vi "UI.vi"(0 "reference in":refnum<class "GUI Setting.lvclass">, 5 "error in (no error)":errorcluster) -> (14 "reference out":refnum<class "GUI Setting.lvclass">, 19 "error out":errorcluster)   [LabVIEW 2019, in "GUI Setting.lvclass"]
uses:
  GUI Setting.lvclass
  D:/GIT H4000/H4000/src/GUI_class/GUI.lvclass
  GUI Settings Indicator.ctl
  GUI_class/GUI.lvclass/GUI.ctl
  d678bd6a-011c-496f-8712-f7d087665a22.vi
  GUI_class/Set Win State.vi
  GUI_class/protected/GetSheredData.vi
  <vilib>/Utility/error.llb/Clear Errors.vi
  ConfigInterface_class/ConfigInterface.lvclass
  GUI_class/GUI.lvclass
  SV_Wrap/SharedVariableWrapper.lvclass
panel:
  in  "GUI Settings Indicator":T1
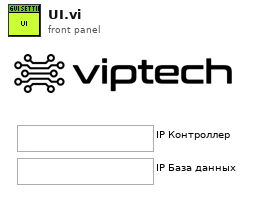
[diagram p1: front panel]
types:
  T1 = typedef "GUI Setting.lvclass/GUI Settings Indicator.ctl" = cluster{"ip_controller":string, "ip_db":string}
  T2 = enum32{"Invalid", "Standard", "Closed", "Hidden", "Minimized", "Maximized"}
  T3 = enum32{"invalid app kind", "Development System", "Run Time System", "Student Edition", "Embedded LabVIEW", "Evaluation", "Custom"}
  T4 = cluster{"Core":cluster{"Current VI Reference":refnum<vi>, "Close Panel on Exit?":bool}, "file settings":string, "GUI Settings Indicator":T1}
  T5 = cluster{"Current VI Reference":refnum<vi>, "Close Panel on Exit?":bool}
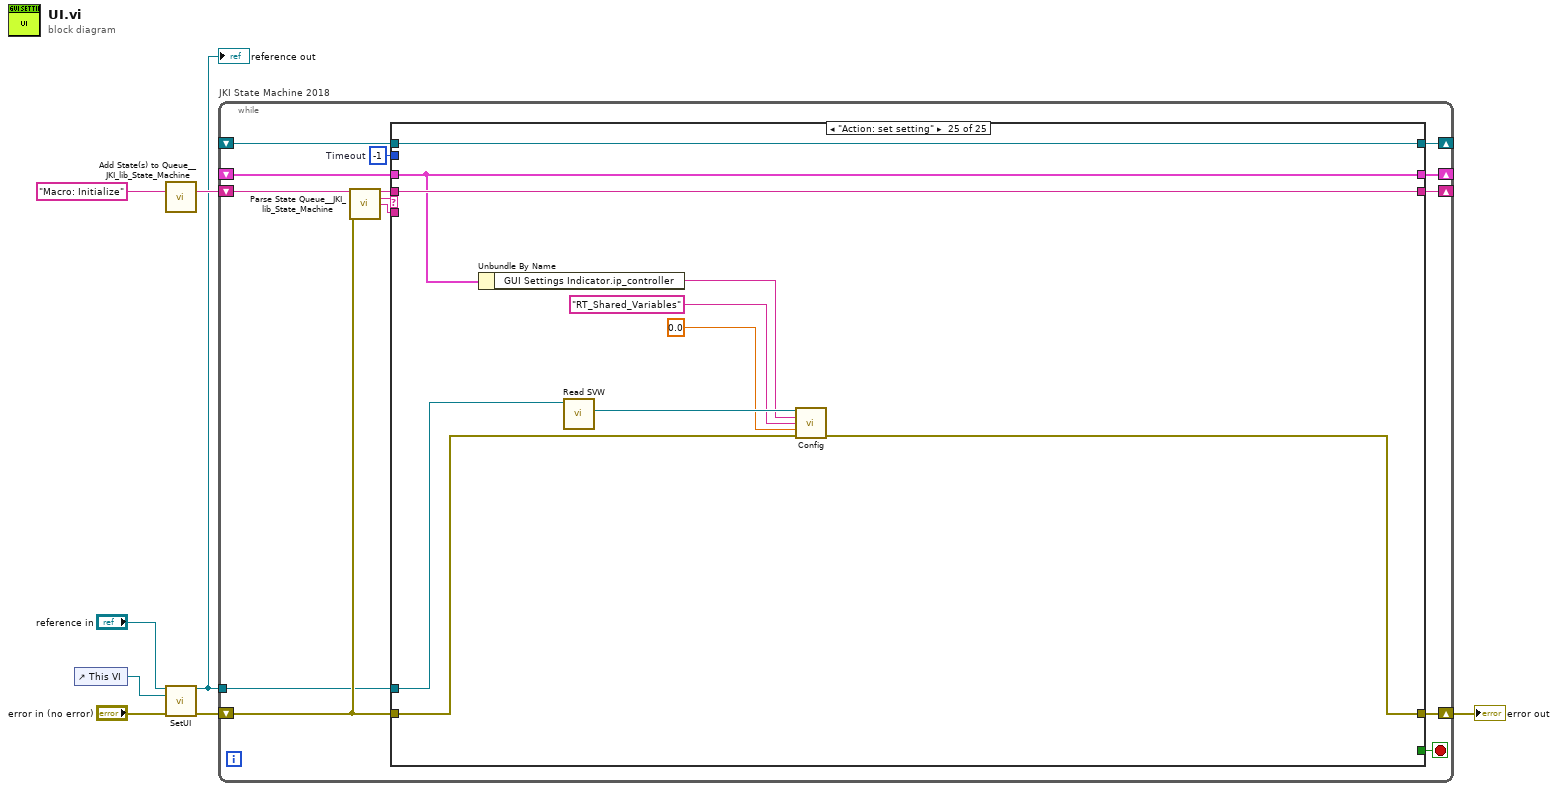
[diagram p0: block diagram]
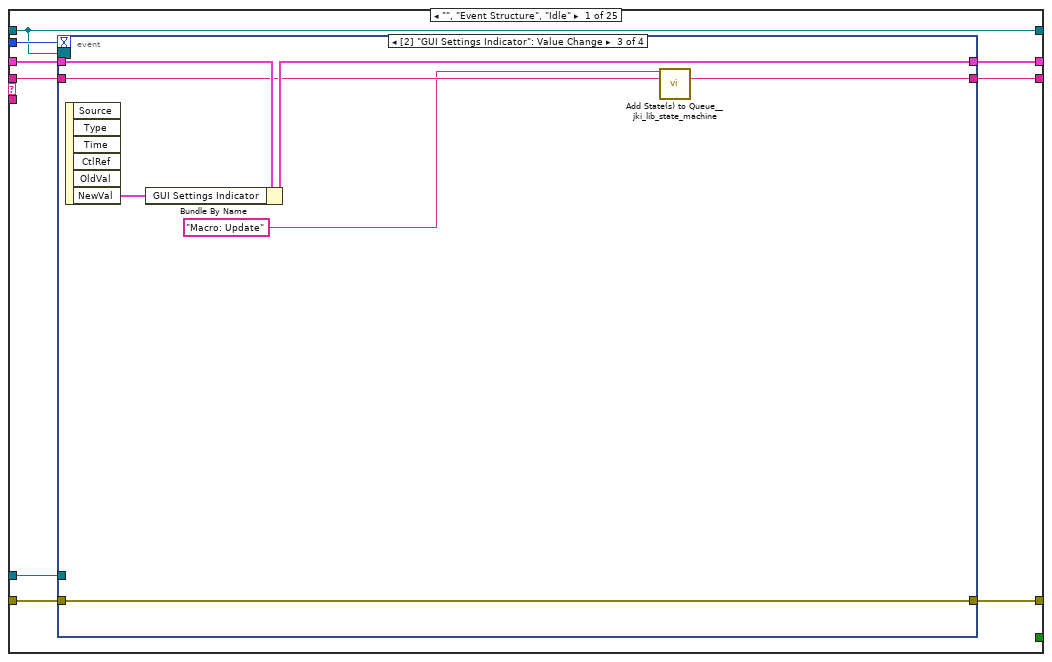
[diagram p2: hidden frame]
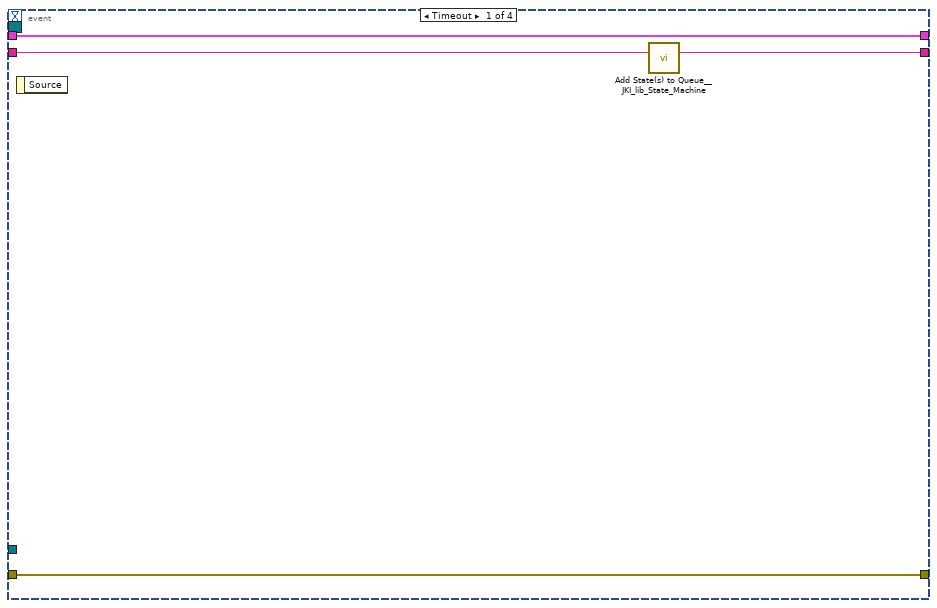
[diagram p3: hidden frame]
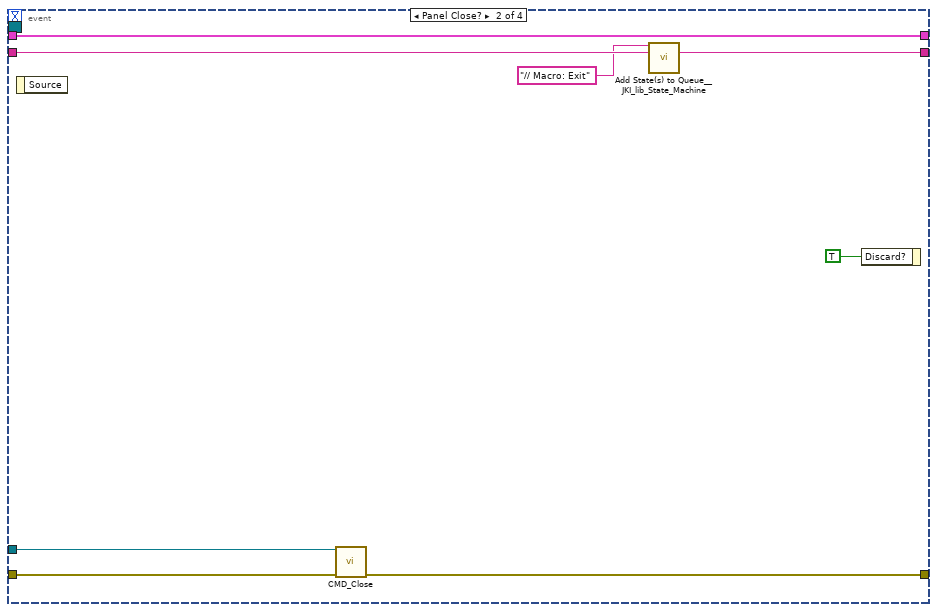
[diagram p4: hidden frame]
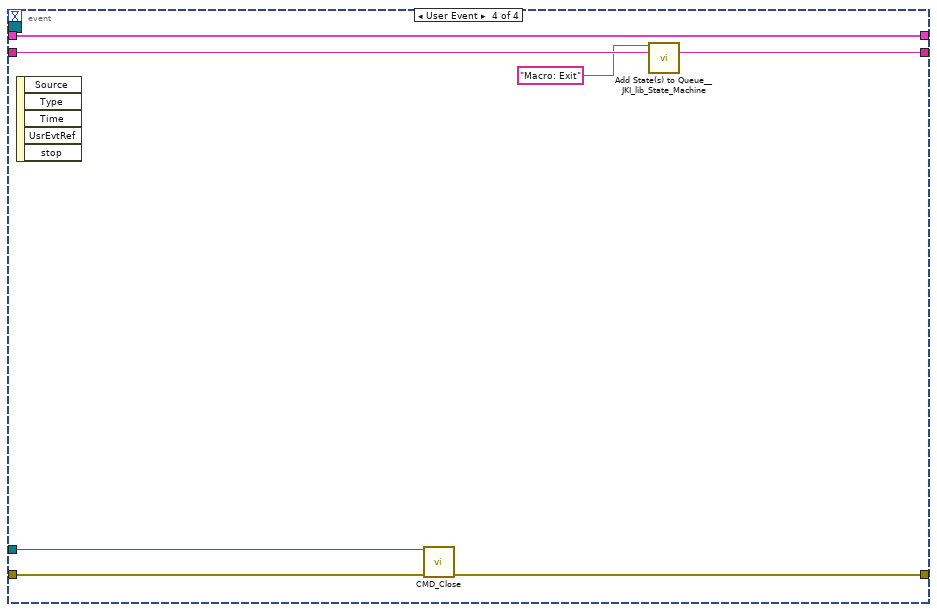
[diagram p5: hidden frame]
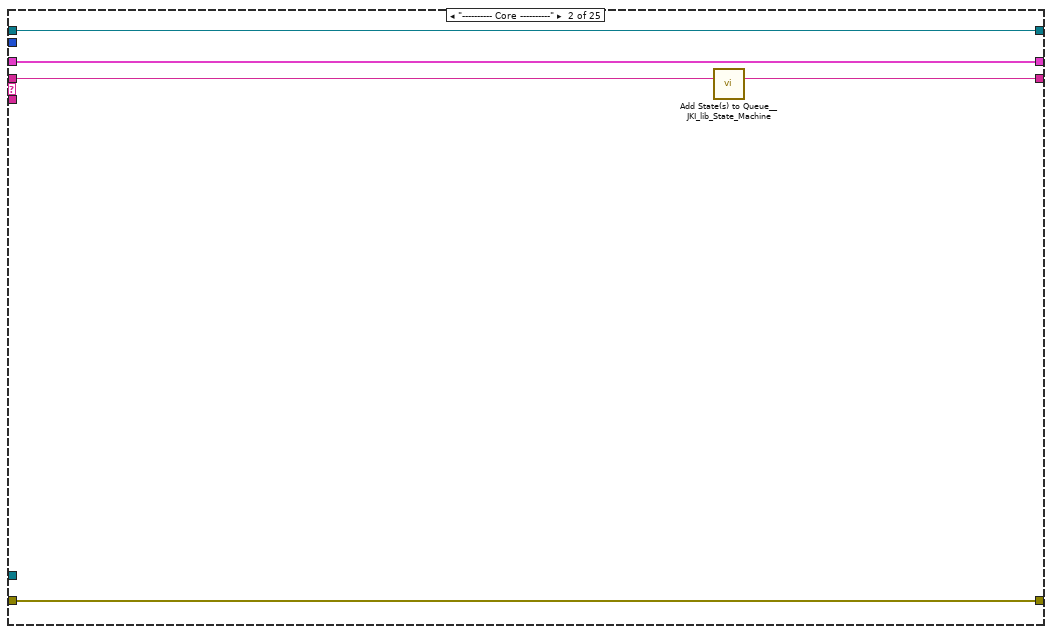
[diagram p6: hidden frame]
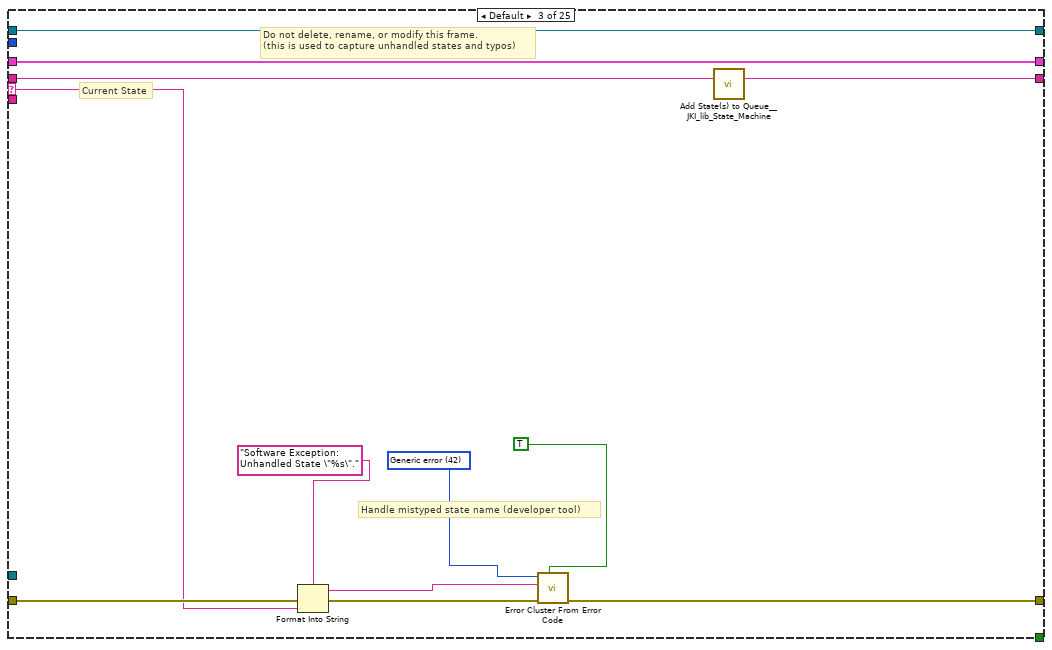
[diagram p7: hidden frame]
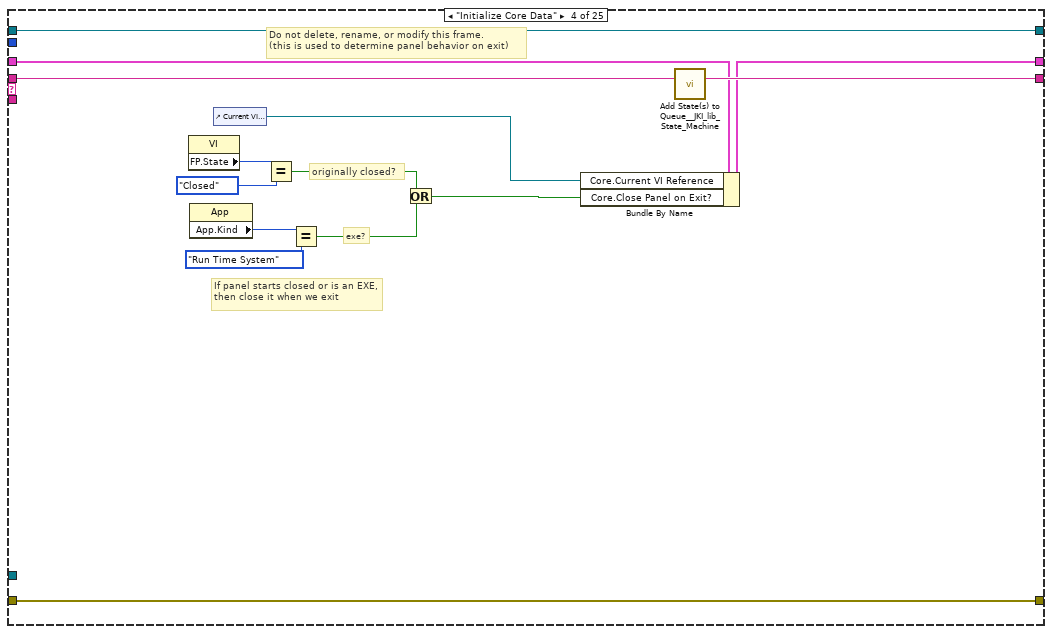
[diagram p8: hidden frame]
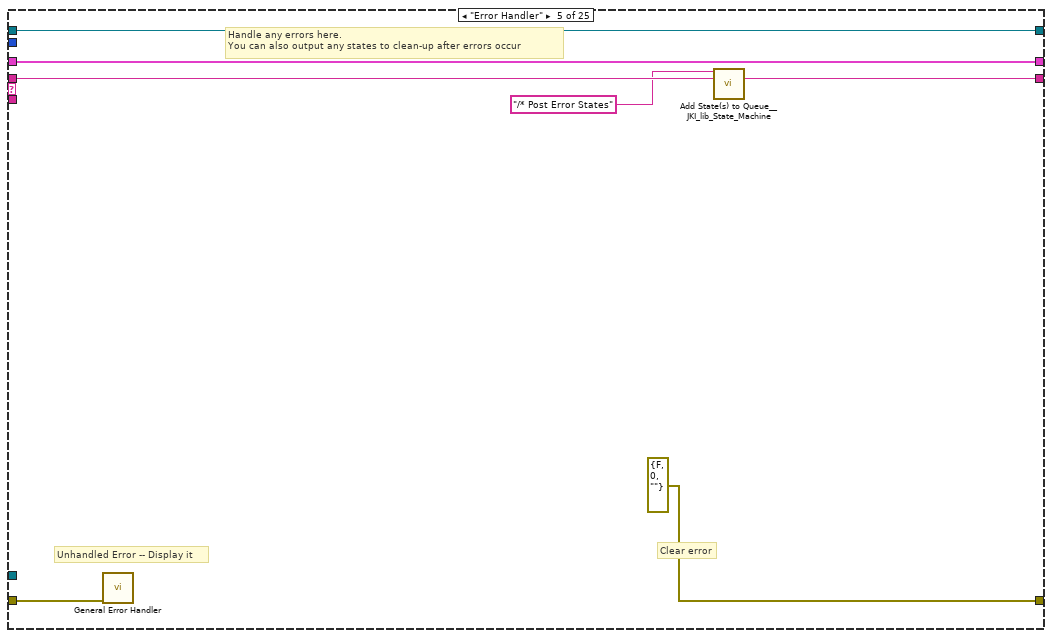
[diagram p9: hidden frame]
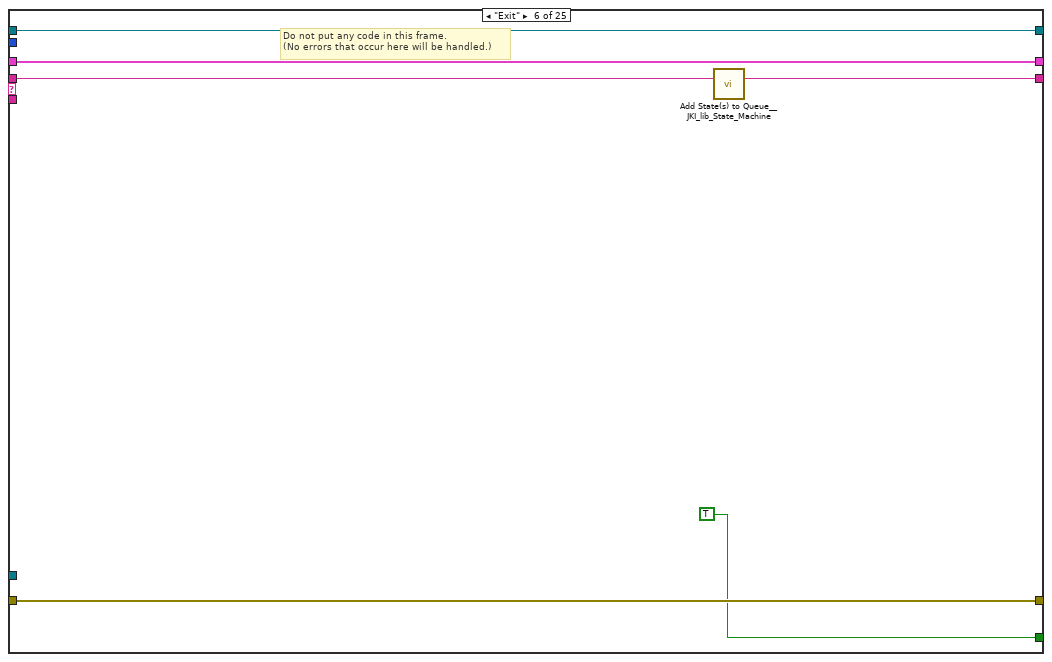
[diagram p10: hidden frame]
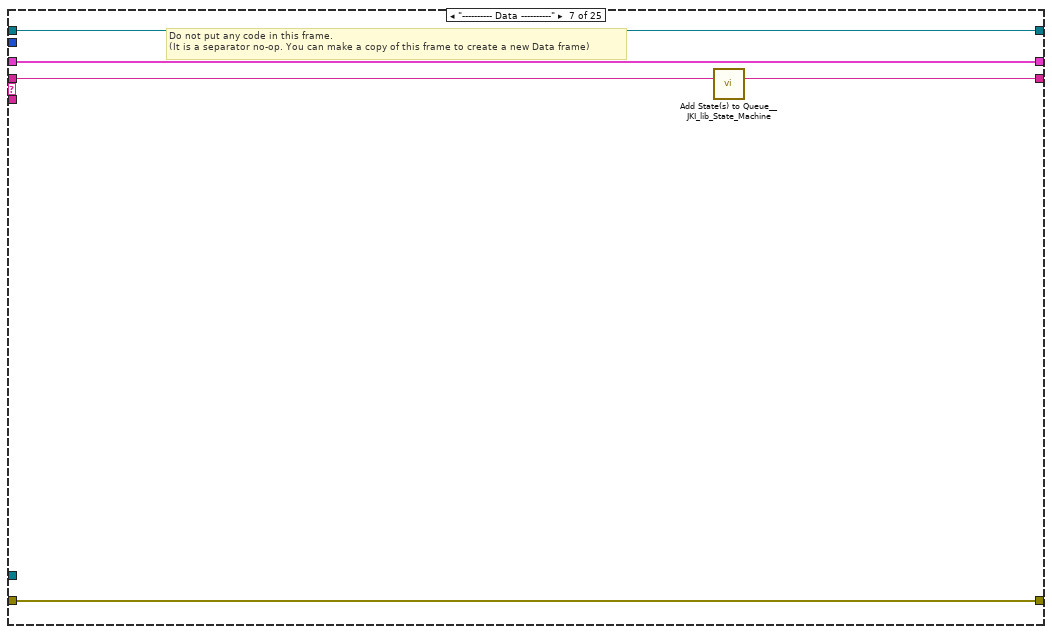
[diagram p11: hidden frame]
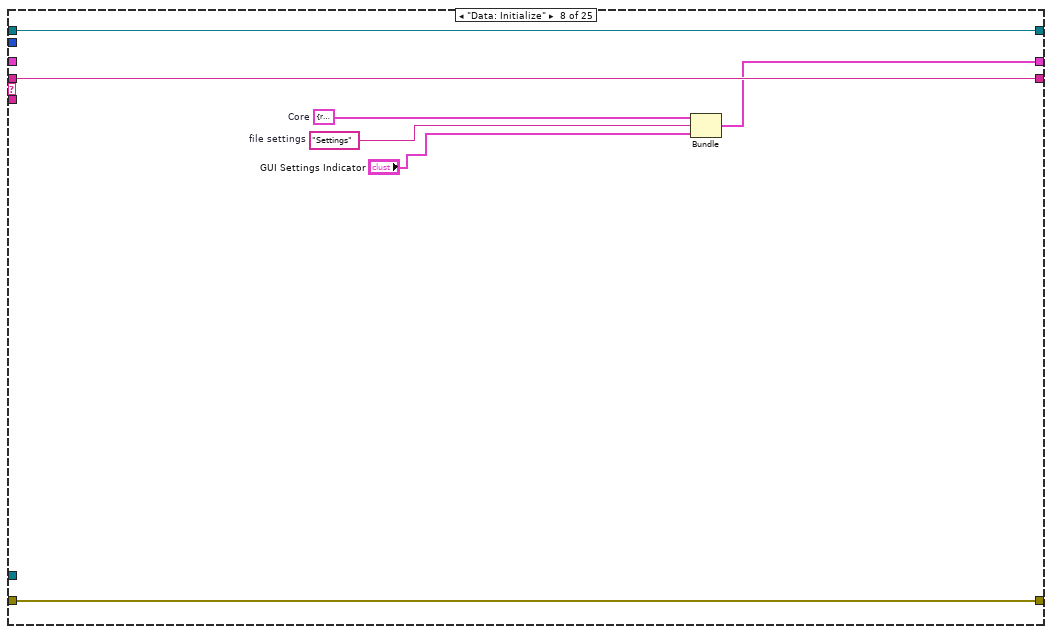
[diagram p12: hidden frame]
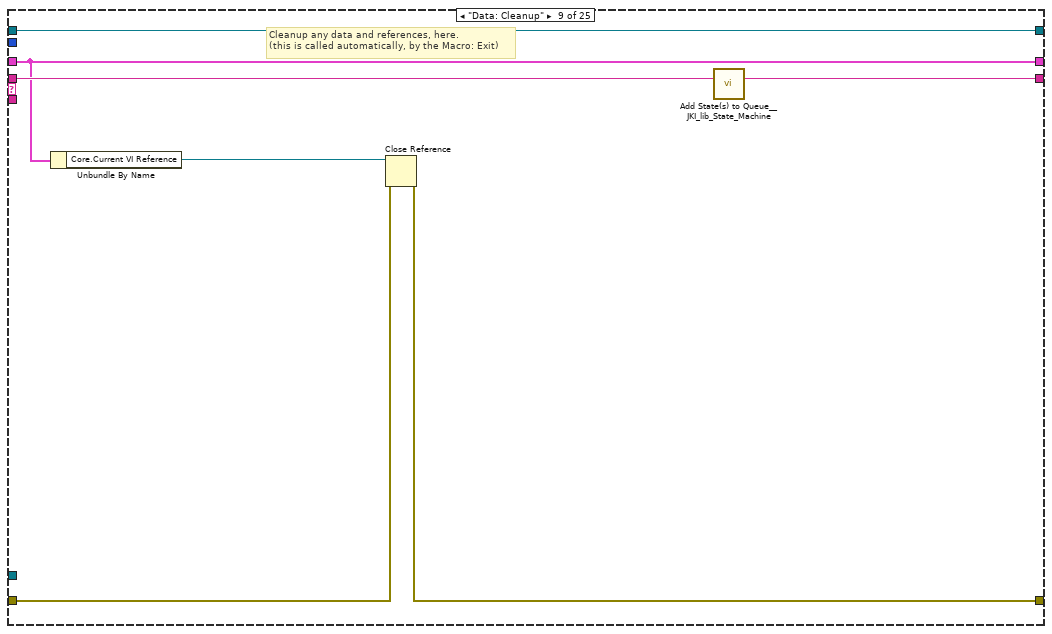
[diagram p13: hidden frame]
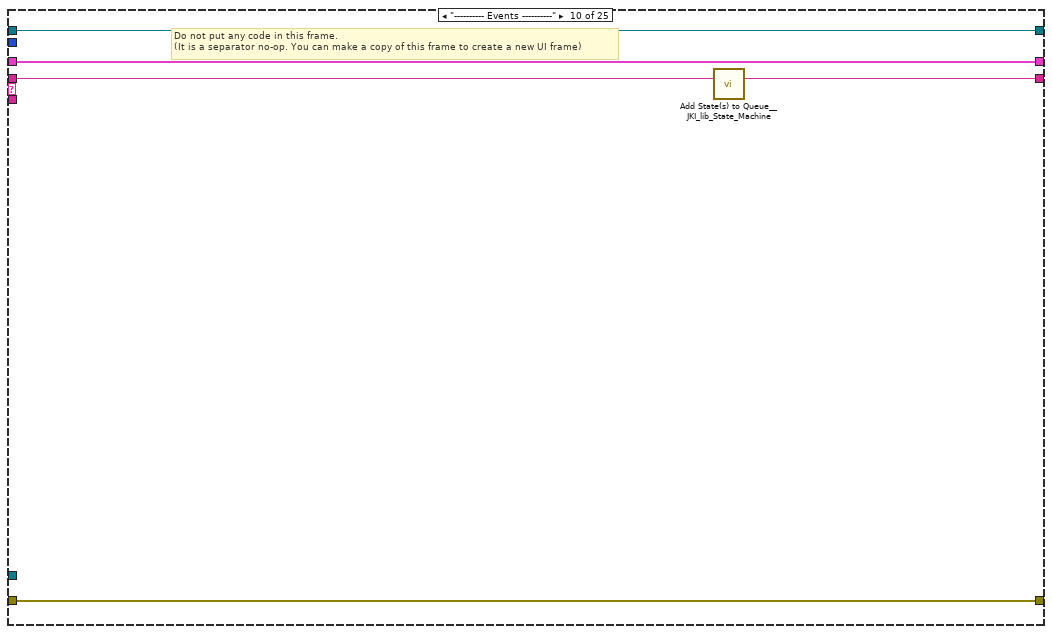
[diagram p14: hidden frame]
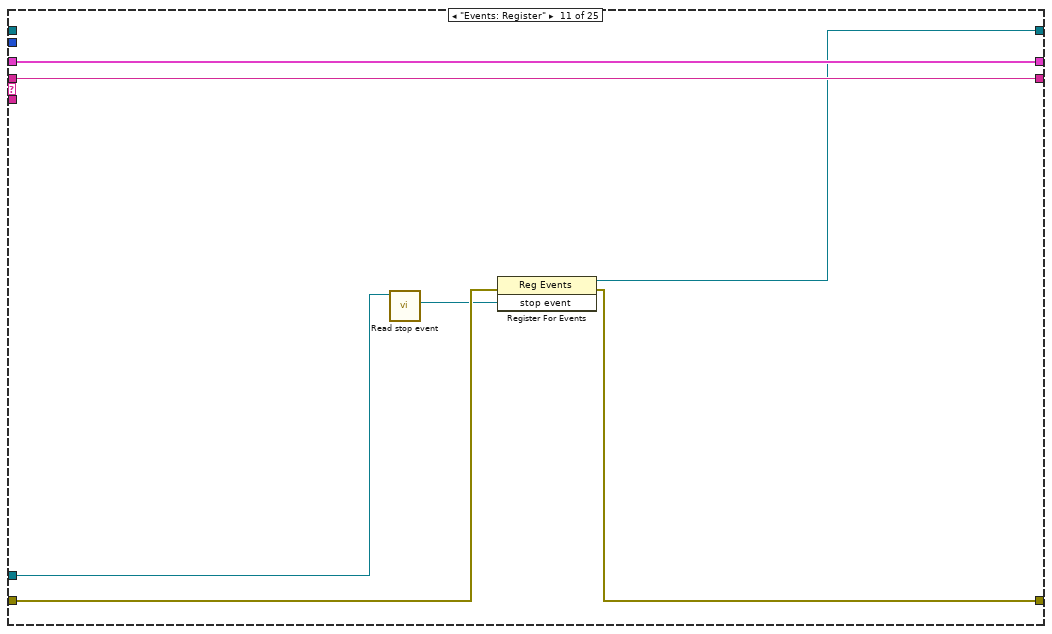
[diagram p15: hidden frame]
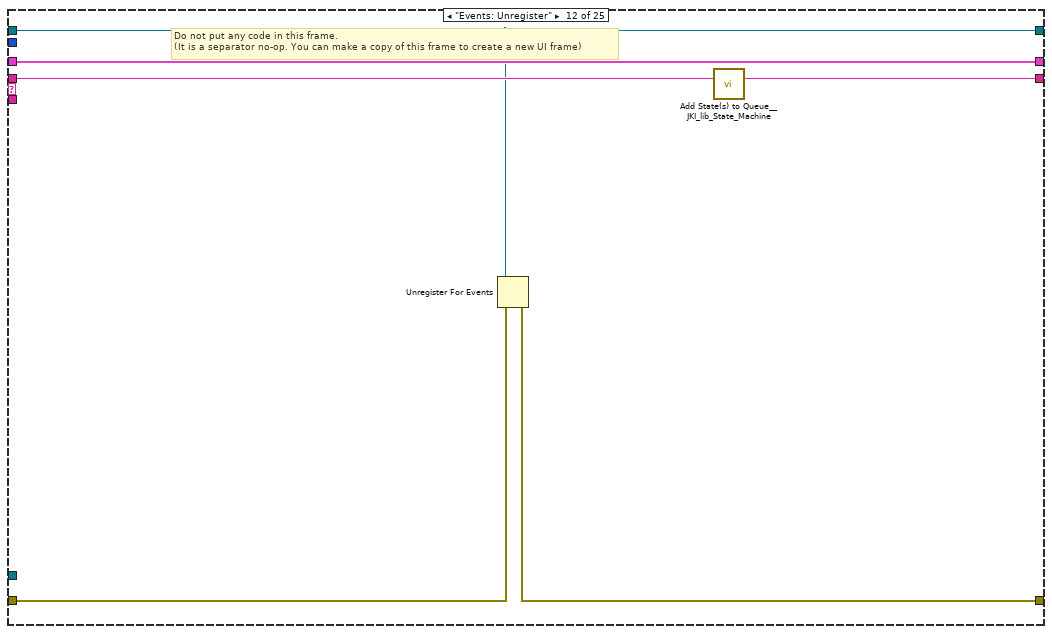
[diagram p16: hidden frame]
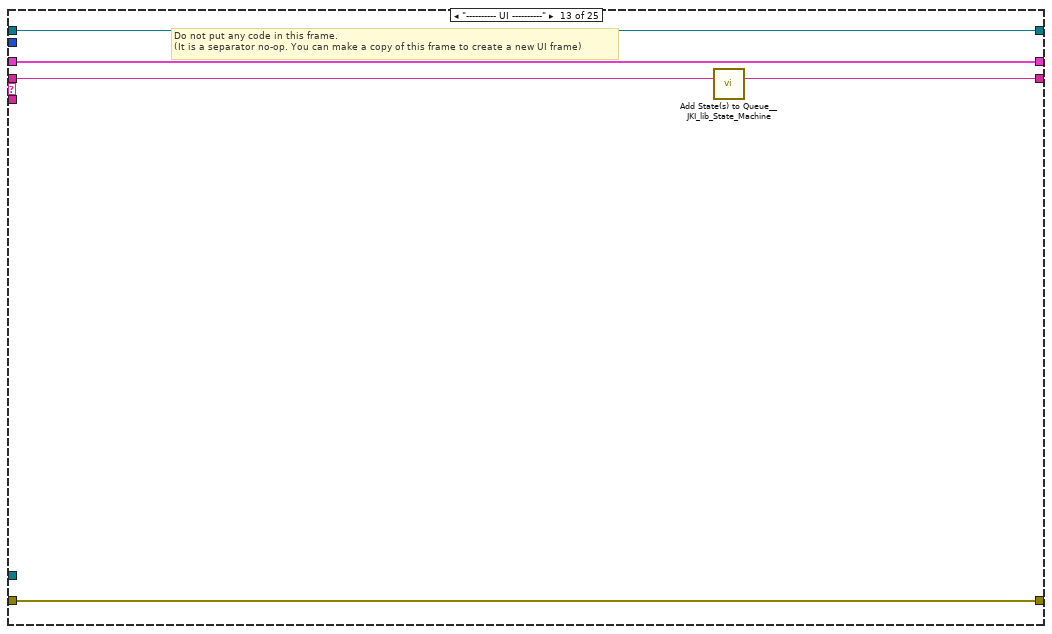
[diagram p17: hidden frame]
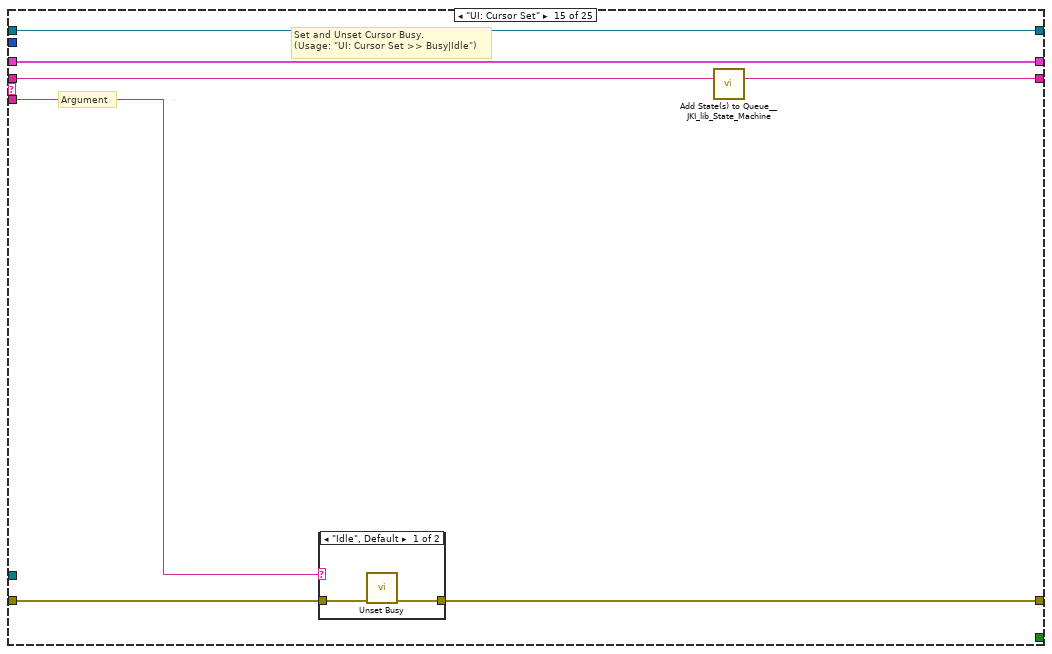
[diagram p19: hidden frame]
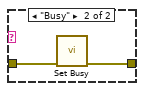
[diagram p20: hidden frame]
diagram:
  n1 = control-ref of="This VI"() -> (w3:refnum<vi>)
  n2 = call <vilib>:"Add State(s) to Queue__JKI_lib_State_Machine.vi"("State(s) in (\"\")"="Macro: Initialize") -> ("States Out"=w8:string)  [unwired: 14 in]
  n3 = call "SetUI.vi"("reference in"="reference in", "UI VI"=w3, "error in (no error)"="error in (no error)") -> ("reference out"=w1:refnum<class "GUI Setting.lvclass">, "error out"=w2:errorcluster)  [unwired: 11 in]
  "reference out" <- w1
  n4 = while "JKI State Machine 2018" {
    shift-right: [w15] -> _
    shift-left: _ -> [w14]
    shift-right: [w18] -> w6
    shift-left: w2 -> [w12]
    shift-right: [w17] -> _
    shift-left: w8 -> [w19]
    tunnel: w1 -> [w11]
    shift-right: [w10] -> _
    shift-left: _ -> [w9]
    stop <- w16 stop-if-true
    w13 = -1  # Timeout
    n5 = call <vilib>:"Parse State Queue__JKI_lib_State_Machine.vi"("State Queue"=w19, "Error In (no error)"=w12) -> ("Remaining States"=w21:string, "Current State"=w22:string, "Arguments"=w20:string)  [unwired: 11 in]
    n6 = case shown="\"Action: set setting\"" w22 {
      selector: w22 -> [_ _ w64 _ _ _ _ _ _ _ _ _ _ _ _ _ _ _ _ _ _ _ _ _ _]
      tunnel: w21 -> [w31 w62 w68 w88 w95 w101 w106 w113 w120 w125 w132 w138 w143 w147 w154 w166 w236 w242 w248 w260 w264 w266 w287 w292 w302]
      tunnel: w20 -> [_ _ _ _ _ _ _ _ _ _ _ _ _ _ w149 w160 _ _ _ _ _ _ _ _ _]
      tunnel: w14 -> [w29 w59 w66 w81 w92 w99 w103 _ w115 w122 w131 w136 w140 w146 w152 w162 w233 w239 w245 w257 w262 w268 w283 w289 w300]
      tunnel: [w28 w60 w70 w85 errorcluster {"status"=FALSE, "code"=0, "source"=""} ("error out") w98 w104 w111 w116 w123 w129 w133 w141 w145 w150 w163 w234 w240 w246 w258 w263 w269 w281 w290 w293] -> w18
      tunnel: w12 -> [w27 w60 w69 w85 w91 w98 w104 w111 w117 w123 w128 w134 w141 w145 w151 w164 w234 w240 w246 w258 w263 w270 w284 w290 w294]
      tunnel: [w30 w61 w67 w87 w94 w100 w105 w113 w119 w124 w132 w137 w142 w147 w153 w165 w235 w241 w247 w259 w264 w266 w287 w292 w302] -> w17
      tunnel: [_ _ _ _ _ TRUE _ _ _ _ _ _ _ _ _ _ _ _ _ _ _ _ _ _ _] -> w16
      tunnel: [w26 w59 w66 w86 w92 w99 w103 w112 w115 w122 w131 w136 w140 w146 w152 w162 w233 w239 w245 w257 w262 w267 w283 w289 w300] -> w15
      tunnel: w13 -> [w25 _ _ _ _ _ _ _ _ _ _ _ _ _ _ _ _ _ _ _ _ _ _ _ _]
      tunnel: w11 -> [w24 _ _ _ _ _ _ _ _ _ w127 _ _ _ _ _ _ _ _ _ _ w271 w285 _ w299]
      tunnel: [w23 w58 w63 w75 w89 w96 w102 w109 w114 w121 w130 w135 w139 w144 w148 w159 w232 w237 w243 w250 w261 w272 w286 w291 w301] -> w10
      tunnel: w9 -> [w23 w58 w63 w75 w89 w96 w102 w109 w114 w121 _ w135 w139 w144 w148 w159 w232 w237 w243 w250 w261 w272 w286 w291 w301]
      frame "", "Event Structure", "Idle" {
        n7 = event shown="[2] \"GUI Settings Indicator\": Value Change" {
          selector: w23 -> [_ _ _ _]
          dyn-events: _ -> [_ _ _ _]
          timeout: w25 -> [_ _ _ _]
          tunnel: w31 -> [w35 w43 w45 w57]
          tunnel: [w34 w42 w46 w56] -> w30
          tunnel: w29 -> [w32 w41 w49 w55]
          tunnel: [w33 w36 w50 w51] -> w28
          tunnel: w27 -> [w33 w37 w50 w52]
          tunnel: [w32 w41 w48 w55] -> w26
          tunnel: w24 -> [_ w38 _ w53]
          event Timeout {
            n8 = event-data() -> ()  [unwired: 1 in, 1 out]
            n9 = call <vilib>:"Add State(s) to Queue__JKI_lib_State_Machine.vi"("State(s) in (\"\")"=w35) -> ("States Out"=w34:string)  [unwired: 14 in]
          }
          event Panel Close? {
            n10 = event-data() -> ()  [unwired: 1 in, 1 out]
            n11 = call "CMD_Close.vi"("reference in"=w38, "error in (no error)"=w37) -> ("error out"=w36:errorcluster)  [unwired: 12 in, 1 out]
            n12 = call <vilib>:"Add State(s) to Queue__JKI_lib_State_Machine.vi"("State(s) in Front (\"\")"="// Macro: Exit", "State(s) in (\"\")"=w43) -> ("States Out"=w42:string)  [unwired: 13 in]
            n13 = event-data("Discard?"=TRUE) -> ()  [unwired: 1 in, 1 out]
          }
          event Value Change {
            n14 = event-data() -> ("NewVal"=w47:T1)  [unwired: 1 in, 5 out]
            n15 = Bundle By Name(cluster=w49, "GUI Settings Indicator"=w47) -> (w48:T4)
            n16 = call <vilib>:"Add State(s) to Queue__jki_lib_state_machine.vi"("State(s) in Front (\"\")"="Macro: Update" ("State(s) in Front (\"\")"), "State(s) in (\"\")"=w45) -> ("States Out"=w46:string)  [unwired: 13 in]
          }
          event User Event {
            n17 = event-data() -> ()  [unwired: 1 in, 5 out]
            n18 = call "CMD_Close.vi"("reference in"=w53, "error in (no error)"=w52) -> ("error out"=w51:errorcluster)  [unwired: 12 in, 1 out]
            n19 = call <vilib>:"Add State(s) to Queue__JKI_lib_State_Machine.vi"("State(s) in Front (\"\")"="Macro: Exit", "State(s) in (\"\")"=w57) -> ("States Out"=w56:string)  [unwired: 13 in]
          }
        }
      }
      frame "---------- Core ----------" {
        n20 = call <vilib>:"Add State(s) to Queue__JKI_lib_State_Machine.vi"("State(s) in (\"\")"=w62) -> ("States Out"=w61:string)  [unwired: 14 in]
      }
      frame Default {
        w73 = 42 items=["No error", "Argument error", "Memory is full", "Out of zone", "End of file", "File already open", "Generic file I/O error", "File not found", "File permission error", "Disk is full", "Duplicate path", "Too many files open", "System feature not enabled", "Resource file not found", "Cannot add resource", "Resource not found", "Image not found", "Image memory error", "Pen does not exist", "Config type invalid", "Config token not found", "Config parse error", "Config memory error", "Bad external code format", "Bad external code offset", "External code not present", "Null window", "Destroy window error", "Null menu", "Print aborted", "Bad print record", "Print driver error", "Windows error during printing", "Memory error during printing", "Print dialog error", "Generic print error", "Invalid device refnum", "Device not found", "Device parameter error", "Device unit error", "Cannot open device", "Device call aborted", "Generic error", "Cancelled by user", "Object ID too low", "Object ID too high", "Object not in heap", "Unknown heap", "Unknown object (invalid DefProc)", "Unknown object (DefProc not in table)", "Message out of range", "Invalid (null) method", "Unknown message", "Manager call not supported", "Bad address", "Network operation in progress", "Network operation timed out", "Connection is busy", "Network attribute not supported", "Network error", "Address in use", "System out of memory", "Connection aborted", "Connection refused", "Not connected", "Already connected", "Connection closed", "Initialization error (interapplication manager)", "Bad occurrence", "Wait on unbound occurrence handler", "Occurrence queue overflow", "Datalog type conflict", "Unused", "Unrecognized type (interapplication manager)", "Memory corrupt", "Failed to make temporary DLL", "Old CIN version", "Drag socket not found", "Failed to load drop-object", "Failed to register OLE object", "Failed to release OLE object", "Format specifier type mismatch", "Unknown format specifier", "Too few format specifiers", "Too many format specifiers", "Scan failed", "Newer CIN version", "Error converting to variant", "Runtime menu error", "Password tampered", "Variant attribute not found", "Incompatible variant data type", "Event data is not available", "Event Store is not present", "Occurrence is not found", "Event Queue is not created", "Event info is not available", "Refnum passed is NULL", "Error retrieving Class GUID", "Error retrieving CoClass GUID", "Error retrieving TypeLib GUID.", "Bad built application magic bytes.", "Specific driver is different from the specific driver associated with the Logical Name.", "There is no session opened to the class driver.", "Max Error", "MAX - Error with config objects", "MAX - Error loading configuration", "MAX - Group not supported"]
        # "Current State"
        # "Do not delete, rename, or modify this frame.\n(this is used to capture unhandled states and typos)"
        # "Handle mistyped state name (developer tool)"
        n21 = Format Into String(format string="Software Exception: Unhandled State \"%s\"." ("message"), error in=w69, w64) -> (resulting string=w72:string, error out=w71:errorcluster)  [unwired: 1 in]
        n22 = call <vilib>:"Error Cluster From Error Code.vi"("show call chain? (False)"=TRUE, "error in (no error)"=w71, "error message (\"\")"=w72, "error code (0)"=w73) -> ("error out"=w70:errorcluster)  [unwired: 5 in]
        n23 = call <vilib>:"Add State(s) to Queue__JKI_lib_State_Machine.vi"("State(s) in (\"\")"=w68) -> ("States Out"=w67:string)  [unwired: 14 in]
      }
      frame "Initialize Core Data" {
        # "Do not delete, rename, or modify this frame.\n(this is used to determine panel behavior on exit)"
        # "originally closed?"
        # "exe?"
        # "If panel starts closed or is an EXE, then close it when we exit"
        n24 = property class="VI"() -> ("FP.State"=w78:T2)  [unwired: 2 in, 2 out]
        n25 = property class="App"() -> ("App.Kind"=w84:T3)  [unwired: 2 in, 2 out]
        n26 = control-ref of="Current VI Reference"() -> (w79:refnum<vi>)
        n27 = Equal?(x=w78, y=T2."Closed" ("Front Panel Window:State")) -> (x = y?=w76:bool)
        n28 = Equal?(x=w84, y=T3."Run Time System" ("Application:Kind")) -> (x = y?=w82:bool)
        n29 = Or(x=w76, y=w82) -> (x .or. y?=w80:bool)
        n30 = Bundle By Name(cluster=w81, "Core.Current VI Reference"=w79, "Core.Close Panel on Exit?"=w80) -> (w86:T4)
        n31 = call <vilib>:"Add State(s) to Queue__JKI_lib_State_Machine.vi"("State(s) in (\"\")"=w88) -> ("States Out"=w87:string)  [unwired: 14 in]
      }
      frame "Error Handler" {
        # "Unhandled Error -- Display it"
        # "Handle any errors here.\nYou can also output any states to clean-up after errors occur"
        # "Clear error"
        n32 = call <vilib>:"General Error Handler.vi"("error in (no error)"=w91) -> ()  [unwired: 10 in, 5 out]
        n33 = call <vilib>:"Add State(s) to Queue__JKI_lib_State_Machine.vi"("State(s) in Front (\"\")"="/* Post Error States", "State(s) in (\"\")"=w95) -> ("States Out"=w94:string)  [unwired: 13 in]
      }
      frame "Exit" {
        # "Do not put any code in this frame.\n(No errors that occur here will be handled.)"
        n34 = call <vilib>:"Add State(s) to Queue__JKI_lib_State_Machine.vi"("State(s) in (\"\")"=w101) -> ("States Out"=w100:string)  [unwired: 14 in]
      }
      frame "---------- Data ----------" {
        # "Do not put any code in this frame.\n(It is a separator no-op. You can make a copy of this frame to create a new Data frame)"
        n35 = call <vilib>:"Add State(s) to Queue__JKI_lib_State_Machine.vi"("State(s) in (\"\")"=w106) -> ("States Out"=w105:string)  [unwired: 14 in]
      }
      frame "Data: Initialize" {
        w108 = "Settings"  # file settings
        w110 = T5 {"Current VI Reference"=refnum, "Close Panel on Exit?"=FALSE}  # Core
        n36 = Bundle("Core"=w110, "file settings"=w108, "GUI Settings Indicator"="GUI Settings Indicator") -> (w112:T4)  [unwired: 1 in]
      }
      frame "Data: Cleanup" {
        # "Cleanup any data and references, here.\n(this is called automatically, by the Macro: Exit)"
        n37 = Unbundle By Name(w115) -> ("Core.Current VI Reference"=w118:refnum<vi>)
        n38 = Close Reference(reference=w118, error in (no error)=w117) -> (error out=w116:errorcluster)
        n39 = call <vilib>:"Add State(s) to Queue__JKI_lib_State_Machine.vi"("State(s) in (\"\")"=w120) -> ("States Out"=w119:string)  [unwired: 14 in]
      }
      frame "---------- Events ----------" {
        # "Do not put any code in this frame.\n(It is a separator no-op. You can make a copy of this frame to create a new UI frame)"
        n40 = call <vilib>:"Add State(s) to Queue__JKI_lib_State_Machine.vi"("State(s) in (\"\")"=w125) -> ("States Out"=w124:string)  [unwired: 14 in]
      }
      frame "Events: Register" {
        n41 = call "Read stop event.vi"("GUI in"=w127) -> ("stop event"=w126:refnum<user-event>)  [unwired: 8 in, 2 out]
        n42 = register-events(error in=w128, w126) -> (reference out=w130:refnum<event-registration>, error out=w129:errorcluster)  [unwired: 1 in]
      }
      frame "Events: Unregister" {
        # "Do not put any code in this frame.\n(It is a separator no-op. You can make a copy of this frame to create a new UI frame)"
        n43 = Unregister For Events(event registration refnum=w135, error in=w134) -> (error out=w133:errorcluster)
        n44 = call <vilib>:"Add State(s) to Queue__JKI_lib_State_Machine.vi"("State(s) in (\"\")"=w138) -> ("States Out"=w137:string)  [unwired: 14 in]
      }
      frame "---------- UI ----------" {
        # "Do not put any code in this frame.\n(It is a separator no-op. You can make a copy of this frame to create a new UI frame)"
        n45 = call <vilib>:"Add State(s) to Queue__JKI_lib_State_Machine.vi"("State(s) in (\"\")"=w143) -> ("States Out"=w142:string)  [unwired: 14 in]
      }
      frame "UI: Initialize" {
      }
      frame "UI: Cursor Set" {
        # "Argument"
        # "Set and Unset Cursor Busy.\n(Usage: \"UI: Cursor Set >> Busy|Idle\")"
        n46 = case shown="\"Idle\", Default" w149 {
          tunnel: w151 -> [w156 w158]
          tunnel: [w155 w157] -> w150
          frame "Idle", Default {
            n47 = call <vilib>:"Unset Busy.vi"("error in (no error)"=w156) -> ("error out"=w155:errorcluster)  [unwired: 10 in]
          }
          frame "Busy" {
            n48 = call <vilib>:"Set Busy.vi"("error in (no error)"=w158) -> ("error out"=w157:errorcluster)  [unwired: 9 in, 1 out]
          }
        }
        n49 = call <vilib>:"Add State(s) to Queue__JKI_lib_State_Machine.vi"("State(s) in (\"\")"=w154) -> ("States Out"=w153:string)  [unwired: 14 in]
      }
      frame "UI: Front Panel State" {
        # "Argument"
        # "Set Front Panel Open or Closed\n(Usage: \"UI: Front Panel State >> Open|Close\")"
        n50 = Unbundle By Name(w162) -> ("Core.Current VI Reference"=w161:refnum<vi>)
        n51 = case shown="\"Minimize\", \"Minimized\"" w160 {
          tunnel: w164 -> [w172 w187 w198 w211 w224]
          tunnel: [w174 w188 w200 w213 w226] -> w163
          tunnel: w161 -> [w173 w185 w199 w212 w225]
          frame "Open", "Standard", Default {
            w167 = T2."Standard" ("State")
            n52 = property class="VI"(reference=w173, error in=w172) -> (reference out=w170:refnum<vi>, error out=w171:errorcluster, "FP.State"=w169:T2)
            n53 = Not Equal?(x=w169, y=w167) -> (x != y?=w168:bool)
            n54 = case shown="True" w168 {
              tunnel: [w178 w180] -> w174
              tunnel: w171 -> [w177 w180]
              tunnel: w170 -> [w176 _]
              tunnel: w167 -> [w175 _]
              frame True {
                n55 = invoke class="VI" method="FP.Open"(reference=w176, error in=w177, "Activate"=TRUE, "State"=w175) -> (error out=w178:errorcluster)  [unwired: 1 in, 4 out]
              }
              frame False {
              }
            }
          }
          frame "Close", "Closed" {
            n56 = property class="VI"(reference=w185, error in=w187) -> (reference out=w184:refnum<vi>, error out=w186:errorcluster, "FP.State"=w182:T2)
            n57 = Not Equal?(x=w182, y=T2."Closed" ("Front Panel Window:State")) -> (x != y?=w181:bool)
            n58 = case shown="True" w181 {
              tunnel: [w189 w192] -> w188
              tunnel: w186 -> [w189 w191]
              tunnel: w184 -> [_ w190]
              frame False {
              }
              frame True {
                n59 = invoke class="VI" method="FP.Close"(reference=w190, error in=w191) -> (error out=w192:errorcluster)  [unwired: 1 in, 2 out]
              }
            }
          }
          frame "Hidden", "Hide" {
            w193 = T2."Hidden" ("State")
            n60 = property class="VI"(reference=w199, error in=w198) -> (reference out=w196:refnum<vi>, error out=w197:errorcluster, "FP.State"=w195:T2)
            n61 = Not Equal?(x=w195, y=w193) -> (x != y?=w194:bool)
            n62 = case shown="True" w194 {
              tunnel: [w204 w205] -> w200
              tunnel: w197 -> [w203 w205]
              tunnel: w196 -> [w202 _]
              tunnel: w193 -> [w201 _]
              frame True {
                n63 = invoke class="VI" method="FP.Open"(reference=w202, error in=w203, "State"=w201) -> (error out=w204:errorcluster)  [unwired: 2 in, 4 out]
              }
              frame False {
              }
            }
          }
          frame "Minimize", "Minimized" {
            w206 = T2."Minimized" ("State")
            n64 = property class="VI"(reference=w212, error in=w211) -> (reference out=w209:refnum<vi>, error out=w210:errorcluster, "FP.State"=w208:T2)
            n65 = Not Equal?(x=w208, y=w206) -> (x != y?=w207:bool)
            n66 = case shown="True" w207 {
              tunnel: [w217 w218] -> w213
              tunnel: w210 -> [w216 w218]
              tunnel: w209 -> [w215 _]
              tunnel: w206 -> [w214 _]
              frame True {
                n67 = invoke class="VI" method="FP.Open"(reference=w215, error in=w216, "State"=w214) -> (error out=w217:errorcluster)  [unwired: 2 in, 4 out]
              }
              frame False {
              }
            }
          }
          frame "Maximize", "Maximized" {
            w219 = T2."Maximized" ("State")
            n68 = property class="VI"(reference=w225, error in=w224) -> (reference out=w222:refnum<vi>, error out=w223:errorcluster, "FP.State"=w221:T2)
            n69 = Not Equal?(x=w221, y=w219) -> (x != y?=w220:bool)
            n70 = case shown="True" w220 {
              tunnel: [w230 w231] -> w226
              tunnel: w223 -> [w229 w231]
              tunnel: w222 -> [w228 _]
              tunnel: w219 -> [w227 _]
              frame True {
                n71 = invoke class="VI" method="FP.Open"(reference=w228, error in=w229, "State"=w227) -> (error out=w230:errorcluster)  [unwired: 2 in, 4 out]
              }
              frame False {
              }
            }
          }
        }
        n72 = call <vilib>:"Add State(s) to Queue__JKI_lib_State_Machine.vi"("State(s) in (\"\")"=w166) -> ("States Out"=w165:string)  [unwired: 14 in]
      }
      frame "---------- Macro ----------" {
        # "Do not put any code in this frame.\n(It is a separator no-op. You can make a copy of this frame to create a new Macro frame)"
        n73 = call <vilib>:"Add State(s) to Queue__JKI_lib_State_Machine.vi"("State(s) in (\"\")"=w236) -> ("States Out"=w235:string)  [unwired: 14 in]
      }
      frame "Macro: Initialize" {
        n74 = call <vilib>:"Add State(s) to Queue__JKI_lib_State_Machine.vi"("State(s) in Front (\"\")"="Data: Initialize\nInitialize Core Data\nEvents: Register\nUI: Initialize\n// UI: Front Panel State >> Open\n\n\nAction: Read Config\n\nMacro: Update\n", "State(s) in (\"\")"=w242) -> ("States Out"=w241:string)  [unwired: 13 in]
      }
      frame "Macro: Update" {
        n75 = call <vilib>:"Add State(s) to Queue__JKI_lib_State_Machine.vi"("State(s) in Front (\"\")"="Action: Update Indicators\nAction: set setting\nAction: Write Config\n", "State(s) in (\"\")"=w248) -> ("States Out"=w247:string)  [unwired: 13 in]
      }
      frame "Macro: Exit" {
        n76 = Unbundle By Name(w257) -> ("Core.Close Panel on Exit?"=w256:bool)
        n77 = Select(t="UI: Front Panel State >> Close", s=w256, f="") -> (s? t:f=w253:string)
        n78 = call <vilib>:"Add State(s) to Queue__JKI_lib_State_Machine.vi"("State(s) in Front (\"\")"="Macro: Update", "State(s) in (\"\")"=w253, "State(s) at Back (\"\")"="Data: Cleanup\nEvents: Unregister\nExit") -> ("States Out"=w251:string)  [unwired: 12 in]
        n79 = call <vilib>:"Add State(s) to Queue__JKI_lib_State_Machine.vi"("State(s) in Front (\"\")"=w251, "State(s) in (\"\")"=w260) -> ("States Out"=w259:string)  [unwired: 13 in]
      }
      frame "---------- Action ----------" {
      }
      frame "Action: Read Config" {
        n80 = call "Read ConfigInterface.vi"("GUI in"=w271) -> ("ConfigInterface"=w265:refnum<class "ConfigInterface.lvclass">)  [unwired: 9 in, 1 out]
        n81 = in-place {
          in-place-border: w265 -> [w278]
          in-place-border: w270 -> [w277]
          in-place-border: [w276] -> w269
          n82 = in-place-cluster #1(w268) -> ("GUI Settings Indicator"=w275:T1, "file settings"=w273:string)
          n83 = call "ReadOrCreate.vim"("reference in"=w278, "Type and Defaults"=w275, "Name"=w273, "error in (no error)"=w277) -> ("Data"=w274:T1, "error out"=w276:errorcluster)  [unwired: 7 in, 3 out]
          n84 = in-place-cluster #1("GUI Settings Indicator"=w274, "file settings"=w273) -> (w267:T4)
        }
      }
      frame "Action: Write Config" {
        n85 = Unbundle By Name(w283) -> ("GUI Settings Indicator"=w280:T1, "file settings"=w279:string)
        n86 = call "Read ConfigInterface.vi"("GUI in"=w285) -> ("ConfigInterface"=w282:refnum<class "ConfigInterface.lvclass">)  [unwired: 9 in, 1 out]
        n87 = call-dynamic "Write.vi"("reference in"=w282, "Data"=w280, "Name"=w279, "error in (no error)"=w284) -> ("error out"=w281:errorcluster)  [unwired: 8 in, 3 out]
      }
      frame "Action: Update Indicators" {
        n88 = Unbundle By Name(w289) -> ("GUI Settings Indicator"=w288:T1)
        n89 = local write "GUI Settings Indicator"(w288) -> ()
      }
      frame "Action: set setting" {
        n90 = Unbundle By Name(w300) -> ("GUI Settings Indicator.ip_controller"=w297:string)
        n91 = call "Read SVW.vi"("GUI in"=w299) -> ("SharedVariableWrapper.lvclass"=w298:refnum<class "SharedVariableWrapper.lvclass">)  [unwired: 10 in]
        n92 = call "Config.vi"("SharedVariableWrapper in"=w298, "host"=w297, "lib"="RT_Shared_Variables", "update timeout"=0.0, "error in"=w294) -> ("error out"=w293:errorcluster)  [unwired: 9 in, 1 out]
      }
    }
  }
  "error out" <- w6
